vi "Done Processing.vi"(8 "error in (no error)":errorcluster, 9 "Notification Message Queue":refnum<queue>, 10 "Internal Message Queue":refnum<queue>) -> (0 "error out":errorcluster)   [LabVIEW 2023, in "HAF.lvlib" / "TestProcessor.lvclass"]
doc: "Signal the Done Event so that the Framework starts the processing shutdown cleanly. Put a Done Message on the Notification Queue so the application knows processing has done too."
uses:
  TestProcessor.lvclass
  Message.ctl
  All Notification Message Ids.ctl
  All Internal Message Ids.ctl
  HAF.lvlib
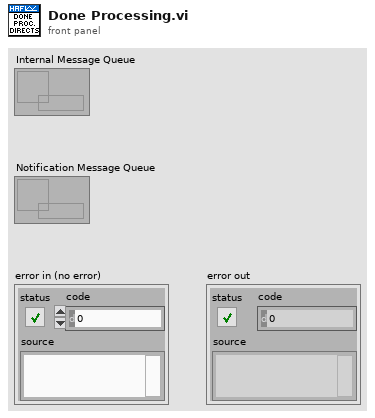
[diagram p1: front panel]
types:
  T1 = typedef "HAF.lvlib/All Internal Message Ids.ctl" = cluster{"Initialise":string, "Process":string, "Continue":string, "Done":string, "Pause":string, "Resume":string, "Stop":string, "Exit":string, "Inject":string}
  T2 = typedef "HAF.lvlib/All Notification Message Ids.ctl" = cluster{"Initialise":string, "Exit":string, "Error":string, "Result":string, "Done":string}
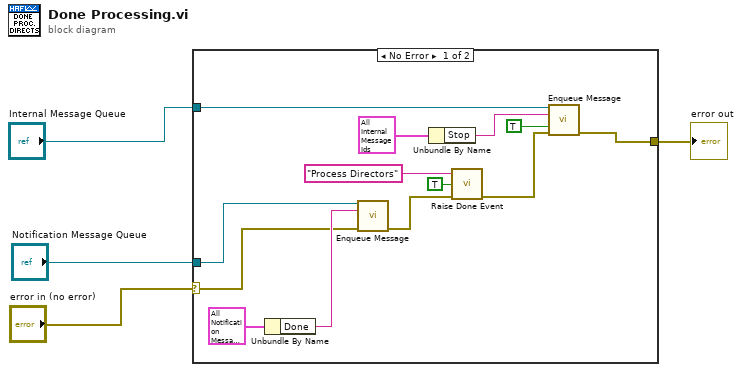
[diagram p0: block diagram]
diagram:
  n1 = case shown="No Error" "error in (no error)" {
    selector: "error in (no error)" -> [w5 w18]
    tunnel: [w17 w18] -> w4
    tunnel: "Internal Message Queue" -> [w14 _]
    tunnel: "Notification Message Queue" -> [w6 _]
    frame No Error {
      n2 = Unbundle By Name(T2 {"Initialise"="Initialise", "Exit"="Exit", "Error"="Error", "Result"="Result", "Done"="Done"} ("Message IDs")) -> ("Done"=w8:string)
      n3 = call "Enqueue Message.vi"("Message Queue In"=w6, "Message Id"=w8, "error in (no error)"=w5) -> ("error out"=w11:errorcluster)  [unwired: 11 in, 1 out]
      n4 = Unbundle By Name(T1 {"Initialise"="Initialise", "Process"="Process", "Continue"="Continue", "Done"="Done", "Pause"="Pause", "Resume"="Resume", "Stop"="Stop", "Exit"="Exit", "Inject"=""} ("Message Ids")) -> ("Stop"=w12:string)
      n5 = call "Raise Done Event.vi"("Raiser Name"="Process Directors", "Send Done"=TRUE, "error in (no error)"=w11) -> ("error out"=w15:errorcluster)  [unwired: 12 in]
      n6 = call "Enqueue Message.vi"("Message Queue In"=w14, "Message Id"=w12, "Priority"=TRUE, "error in (no error)"=w15) -> ("error out"=w17:errorcluster)  [unwired: 10 in, 1 out]
    }
    frame Error {
    }
  }
  "error out" <- w4
